vi "solar_misc Parse WSV.vi"(0 "WSV String":string) -> (6 "2D Array":string[][](array[string]))   [LabVIEW 2018]
doc: "This parses a whitespace separated value table into a 2d array. Whitespace may include spaces and tabs. Line feeds and carriage returns are considered separate rows."
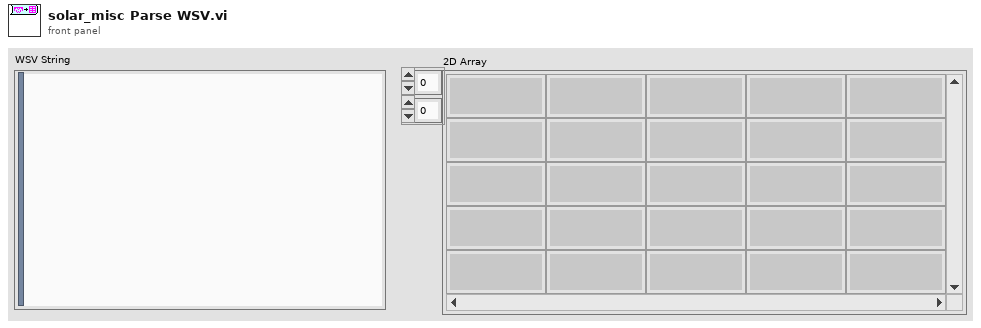
[diagram p1: front panel]
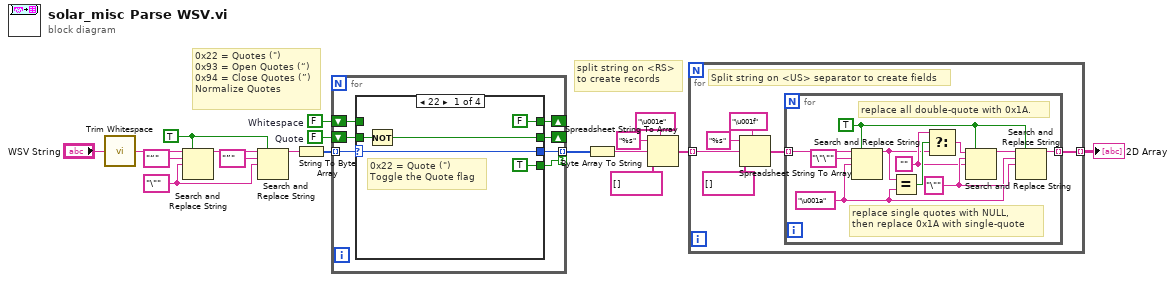
[diagram p0: block diagram]
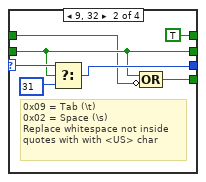
[diagram p2: hidden frame]
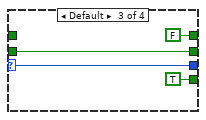
[diagram p3: hidden frame]
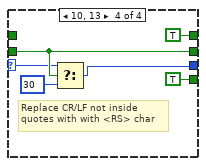
[diagram p4: hidden frame]
diagram:
  w1 = FALSE  # Whitespace
  w13 = FALSE  # Quote
  w14 = TRUE ("replace all? (F)")
  w16 = "\"" ("replace string (\"\")")
  # "split string on <RS>\nto create records"
  # "0x22 = Quotes (\")\n0x93 = Open Quotes (“)\n0x94 = Close Quotes (”)\nNormalize Quotes"
  n1 = call <vilib>:"Trim Whitespace.vi"("string"="WSV String") -> ("trimmed string"=w3:string)  [unwired: 1 in]
  n2 = Search and Replace String(replace all?=w14, input string=w3, search string="“", replace string=w16) -> (result string=w17:string)  [unwired: 1 in, 6 out]
  n3 = Search and Replace String(replace all?=w14, input string=w17, search string="”", replace string=w16) -> (result string=w10:string)  [unwired: 1 in, 6 out]
  n4 = String To Byte Array(string=w10) -> (unsigned byte array=w12:u8[])
  n5 = for {
    tunnel: w12 -> [w22] mode=indexing
    shift-right: [w24] -> _
    shift-left: w13 -> [w25]
    tunnel: [w23] -> w11 mode=indexing if=w19
    shift-right: [w21] -> _
    shift-left: w1 -> [w20]
    n6 = case shown="22" w22 {
      selector: w22 -> [w29 w37 w40 w44]
      tunnel: w25 -> [w28 w34 w41 w47]
      tunnel: [w30 w34 w41 w47] -> w24
      tunnel: [w29 w35 w40 w45] -> w23
      tunnel: w20 -> [_ w33 _ _]
      tunnel: [FALSE ("Whitespace") TRUE ("Whitespace") FALSE ("Whitespace") TRUE ("Whitespace")] -> w21
      tunnel: [TRUE w32 TRUE TRUE] -> w19
      frame 34 {
        # "0x22 = Quote (\")\nToggle the Quote flag"
        n7 = Not(x=w28) -> (.not. x?=w30:bool)
      }
      frame 9, 32 {
        # "0x09 = Tab (\\t)\n0x02 = Space (\\s)\nReplace whitespace not inside \nquotes with with <US> char"
        n8 = Select(t=w37, s=w34, f=u8 31) -> (s? t:f=w35:u8)
        n9 = Compound Arithmetic op=OR(w34, invert w33) -> (w32:bool)
      }
      frame Default {
      }
      frame 10, 13 {
        # "Replace CR/LF not inside \nquotes with with <RS> char"
        n10 = Select(t=w44, s=w47, f=u8 30) -> (s? t:f=w45:u8)
      }
    }
  }
  n11 = Byte Array To String(unsigned byte array=w11) -> (string=w2:string)
  n12 = Spreadsheet String To Array(delimiter (Tab)="\u001e", format string="%s", spreadsheet string=w2, array type (2D Dbl)=string[] []) -> (array=w8:string[])
  n13 = for {
    tunnel: w8 -> [w53] mode=indexing
    tunnel: [w50] -> w5 mode=indexing
    # "Split string on <US> separator to create fields"
    n14 = Spreadsheet String To Array(delimiter (Tab)="\u001f", format string="%s", spreadsheet string=w53, array type (2D Dbl)=string[] []) -> (array=w51:string[])
    n15 = for {
      tunnel: w51 -> [w54] mode=indexing
      tunnel: [w55] -> w50 mode=indexing
      w58 = ""
      w61 = "\"" ("input string")
      w62 = TRUE ("replace all? (F)")
      w60 = "\u001a" ("replace string (\"\")")
      # "replace single quotes with NULL,\nthen replace 0x1A with single-quote"
      # "replace all double-quote with 0x1A."
      n16 = Search and Replace String(replace all?=w62, input string=w54, search string="\"\"", replace string=w60) -> (result string=w57:string)  [unwired: 1 in, 6 out]
      n17 = Equal?(x=w57, y=w60) -> (x = y?=w59:bool)
      n18 = Select(t=w58, s=w59, f=w57) -> (s? t:f=w56:string)
      n19 = Search and Replace String(replace all?=w62, input string=w56, search string=w61, replace string=w58) -> (result string=w63:string)  [unwired: 1 in, 6 out]
      n20 = Search and Replace String(replace all?=w62, input string=w63, search string=w60, replace string=w61) -> (result string=w55:string)  [unwired: 2 in, 5 out]
    }
  }
  "2D Array" <- w5
